vi "UI_init_box.vi"(10 "安全报警UI":refnum<vi>) -> (2 "安全报警UI 2":refnum<vi>)   [LabVIEW 2018, in "UI.lvlib"]
uses:
  UI.lvlib
panel:
  in  "位置:置顶":i32
  in  "位置:居左":i32
  in  "边界:区域宽度":u32
  in  "边界:区域高度":u32
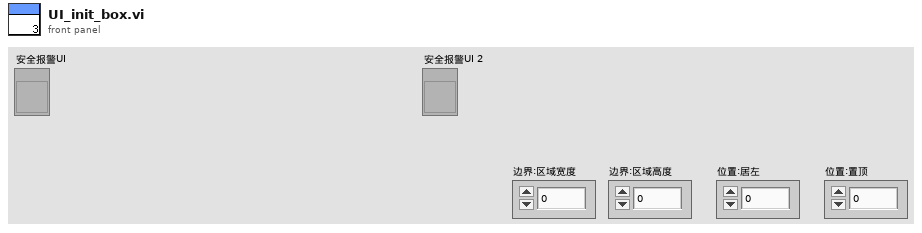
[diagram p1: front panel]
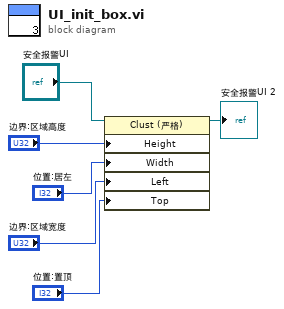
[diagram p0: block diagram]
diagram:
  n1 = property class="Clust (严格)"(reference="安全报警UI", "Height"="边界:区域高度", "Width"="位置:居左", "Left"="边界:区域宽度", "Top"="位置:置顶") -> (reference out=→"安全报警UI 2":refnum<vi>)  [unwired: 1 in, 1 out]
